vi "HMU Cal - Get Cal Tone Power.vi"(5 "Tone Frequency (Hz)":dbl format="%#_6p", 9 "Desired RFout Power (dBm)":dbl=15.0 format="%#_6p", 11 "error in (no error)":errorcluster) -> (10 "Coerced RFout Power (dBm)":dbl, 15 "error out":errorcluster)   [LabVIEW 2023, in "RFFixtureCharact.RFPM.lvlib" / "SG SC2250 Path.lvclass"]
uses:
  SG SC2250 Path.lvclass
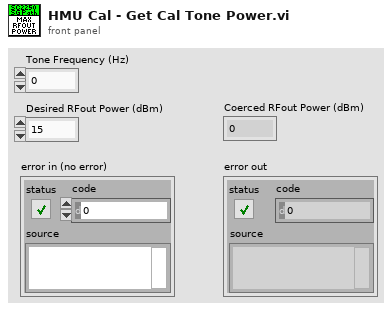
[diagram p1: front panel]
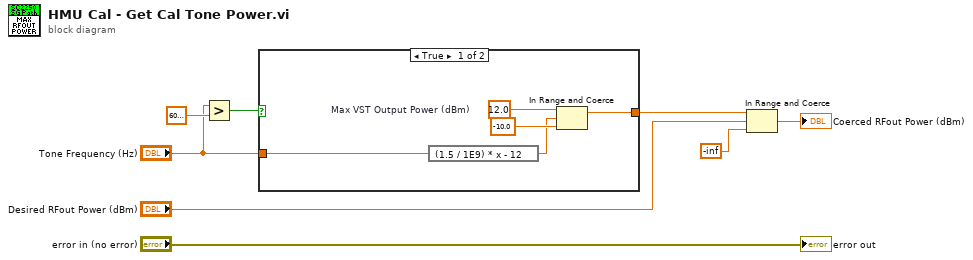
[diagram p0: block diagram]
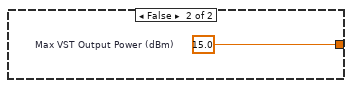
[diagram p2: hidden frame]
diagram:
  n1 = Greater?(x="Tone Frequency (Hz)", y=6000000000.0 ("RF Frequency (Hz)")) -> (0:w6:bool)
  n2 = case shown="True" w6 {
    tunnel: "Tone Frequency (Hz)" -> [w10 _]
    tunnel: [w9 w14] -> w3
    frame True {
      w13 = 12.0  # Max VST Output Power (dBm)
      n3 = expression code="(1.5 / 1E9) * x - 12"(w10) -> (w11:dbl)
      n4 = In Range and Coerce(upper limit=w13, x=w11, lower limit=-10.0) -> (coerced(x)=w9:dbl)  [unwired: 1 out]
    }
    frame False {
      w14 = 15.0  # Max VST Output Power (dBm)
    }
  }
  n5 = In Range and Coerce(upper limit=w3, x="Desired RFout Power (dBm)", lower limit=-inf) -> (coerced(x)=→"Coerced RFout Power (dBm)":dbl)  [unwired: 1 out]
  "error out" <- "error in (no error)"
